vi "SettleDrift.vi"() -> ()   [LabVIEW 2014]
uses:
  <userlib>/Nanonis Prog Interface V5/Nanonis Prog Interface.lvlib
panel:
  out "Y":sgl(graph)
  out "X":sgl(graph)
  in  "Drift correction Pixels":i32
  in  "stop":bool
  in  "Correlate":u16(ring) items=["first Frame", "successive Frames"]
  out "Y Offset":dbl format="%#_6p"
  out "X Offset":dbl format="%#_6p"
  out "X drift":i32
  out "Y drift":i32
  out "Last Drift detected":i32=40
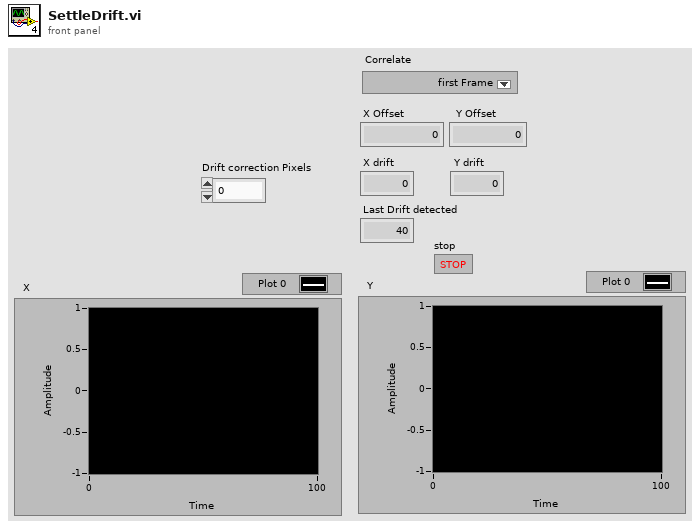
[diagram p1: front panel]
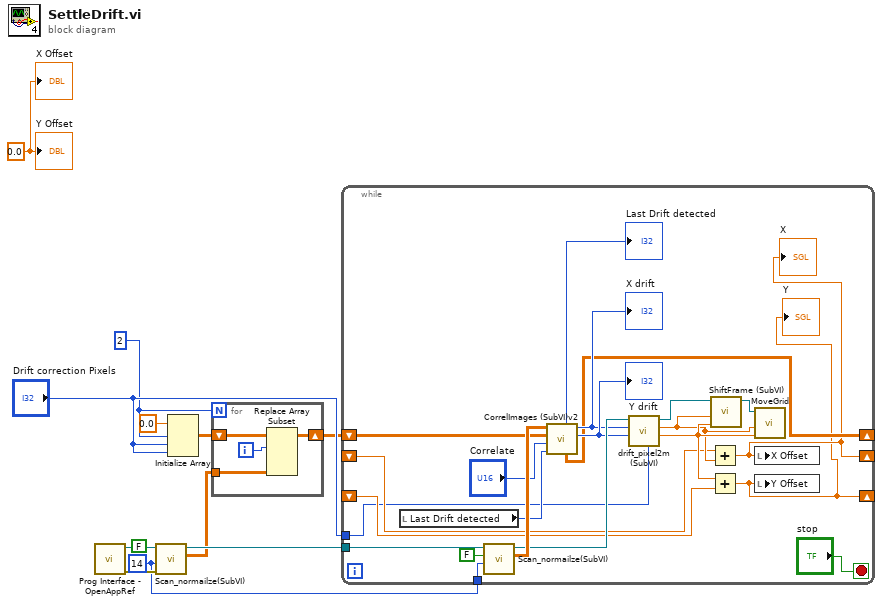
[diagram p0: block diagram]
diagram:
  w2 = u8 14 ("Channel index (0-23)")
  w3 = 2 ("dimension size")
  w9 = 0.0 ("X Offset")
  n1 = call <userlib>:"Prog Interface - OpenAppRef.vi"() -> ("Error out"=w11:errorcluster, "Application reference"=w10:refnum<vi>)  [unwired: 6 in]
  n2 = call "Scan_normailze(SubVI).vi"("error in (no error)"=w11, "Channel index (0-23)"=w2, "Normalization"=FALSE, "Application in"=w10) -> ("Array"=w6:dbl[][], "Application out"=w12:refnum<vi>)  [unwired: 5 in, 1 out]
  n3 = Initialize Array(0.0 ("element"), w3, "Drift correction Pixels", "Drift correction Pixels") -> (w7:dbl[][][])
  n4 = for {
    N: w3 -> [_]
    tunnel: w6 -> [w15]
    shift-right: [w14] -> w4
    shift-left: w7 -> [w16]
    i -> [w13]
    n5 = Replace Array Subset(array=w16, new element=w15, index (dim 0)=w13) -> (w14:dbl[][][])  [unwired: 2 in]
  }
  n6 = while {
    shift-right: [w20] -> _
    shift-left: _ -> [w28]
    shift-right: [w19] -> _
    shift-left: _ -> [w27]
    tunnel: w12 -> [w23]
    shift-right: [w22] -> _
    shift-left: w4 -> [w29]
    tunnel: "Drift correction Pixels" -> [w21]
    tunnel: w2 -> [w18]
    stop <- "stop" stop-if-true
    n7 = local read "Last Drift detected"() -> (w32:i32)
    n8 = call "Scan_normailze(SubVI).vi"("Channel index (0-23)"=w18, "Normalization"=FALSE, "Application in"=w23) -> ("Array"=w38:dbl[][], "Application out"=w30:refnum<vi>)  [unwired: 6 in, 1 out]
    n9 = call "CorrelImages (SubVI)v2.vi"("last drift detected"=w32, "Correlate"="Correlate", "Ref Array"=w29, "New Image"=w38) -> ("Y drift"=w25:i32, "X drift"=w24:i32, "Ref Array out"=w22:dbl[][][], "Queue Steps"=→"Last Drift detected":i32)  [unwired: 4 in]
    "X drift" <- w24
    "Y drift" <- w25
    n10 = call "drift_pixel2m (SubVI).vi"("Application in"=w30, "X drift"=w24, "Y drift"=w25, "Drift correction Pixels"=w21) -> ("Application out"=w36:refnum<vi>, "x drift"=w34:sgl, "y drift"=w35:sgl)  [unwired: 2 in, 1 out]
    n11 = Add(x=w28, y=w34) -> (x+y=w20:sgl)
    "X" <- w20
    n12 = Add(x=w35, y=w27) -> (x+y=w19:sgl)
    "Y" <- w19
    n13 = call "ShiftFrame (SubVI).vi"("Y shift"=w35, "X shift"=w34, "Application in"=w36) -> ("Application out"=w37:refnum<vi>)  [unwired: 8 in]
    n14 = call "MoveGrid.vi"("y"=w35, "x"=w34, "Application ref in"=w37) -> ()  [unwired: 7 in, 2 out]
    n15 = local write "X Offset"(w20) -> ()
    n16 = local write "Y Offset"(w19) -> ()
  }
  "X Offset" <- w9
  "Y Offset" <- w9
